vi "Func1.vi"(8 "error in (no error)":errorcluster, 11 "OperationLogger (proxy) in":refnum<class "OperationLogger (proxy).lvclass">) -> (0 "error out":errorcluster, 3 "OperationLogger (proxy) out":refnum<class "OperationLogger (proxy).lvclass">)   [LabVIEW 2014, in "Normal Proxy.lvlib" / "OperationLogger (proxy).lvclass"]
uses:
  OperationLogger (proxy).lvclass
  OperationLogger (proxy).lvclass/OperationLogger (proxy).ctl
  Subject/Subject.lvclass
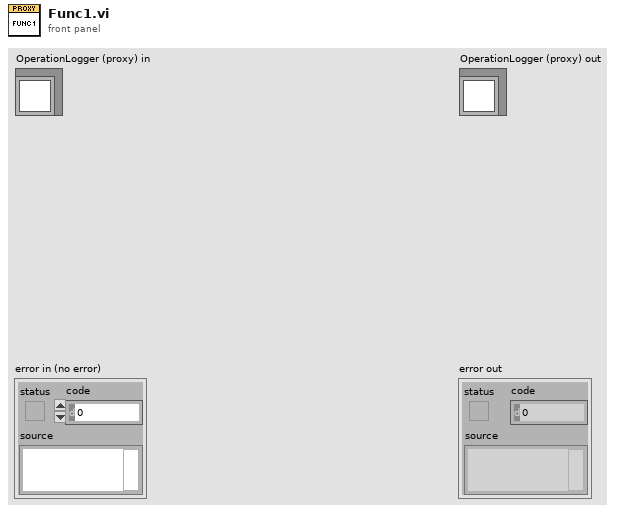
[diagram p1: front panel]
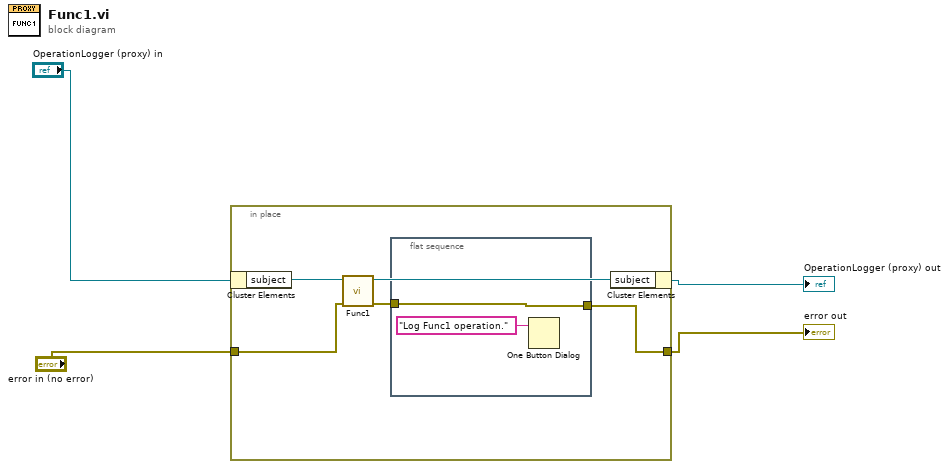
[diagram p0: block diagram]
diagram:
  n1 = in-place {
    in-place-border: "error in (no error)" -> [w7]
    in-place-border: [w6] -> w1
    n2 = in-place-cluster #1("OperationLogger (proxy) in") -> ("subject"=w9:refnum<class "Subject.lvclass">)
    n3 = call-dynamic "Func1.vi"("error in (no error)"=w7, "Subject in"=w9) -> ("error out"=w5:errorcluster, "Subject out"=w8:refnum<class "Subject.lvclass">)  [unwired: 8 in]
    n4 = flat-sequence {
      tunnel: [w11] -> w6
      tunnel: w5 -> [w11]
      frame #0 {
        n5 = One Button Dialog(message="Log Func1 operation.") -> ()  [unwired: 1 in, 1 out]
      }
    }
    n6 = in-place-cluster #1("subject"=w8) -> (→"OperationLogger (proxy) out":refnum<class "OperationLogger (proxy).lvclass">)
  }
  "error out" <- w1
